vi "sub_main_F9P.vi"(8 "error in":errorcluster) -> (0 "error out":errorcluster)   [LabVIEW 2019]
panel:
  out "n":i32
  out "n2":i32
  out "n1":i32
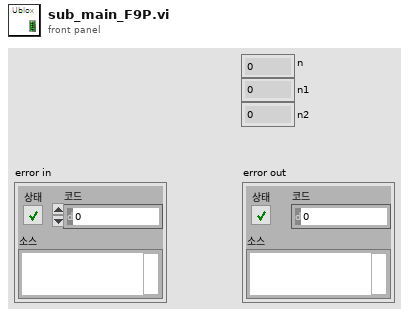
[diagram p1: front panel]
types:
  T1 = enum16{"GxDTM", "GxGBS", "GxGGA", "GxGLL", "GxGNS", "GxGRS", "GxGSA", "GxGST", "GxGSV", "GxRLM", "GxRMC", "GxTHS", "GxTXT", "GxVLW", "GxVTG", "GxZDA"}
  T2 = typedef "error_cluster.ctl" = cluster{"AGV":u8, "AGV Estop":u8, "Obstacle":u8, "Heading":u8, "Waypt":u8, "GNSS":u8, "VLP16":u8, "Cam":u8, "RPLidar":u8, "Joystick":u8, "IMU":u8}
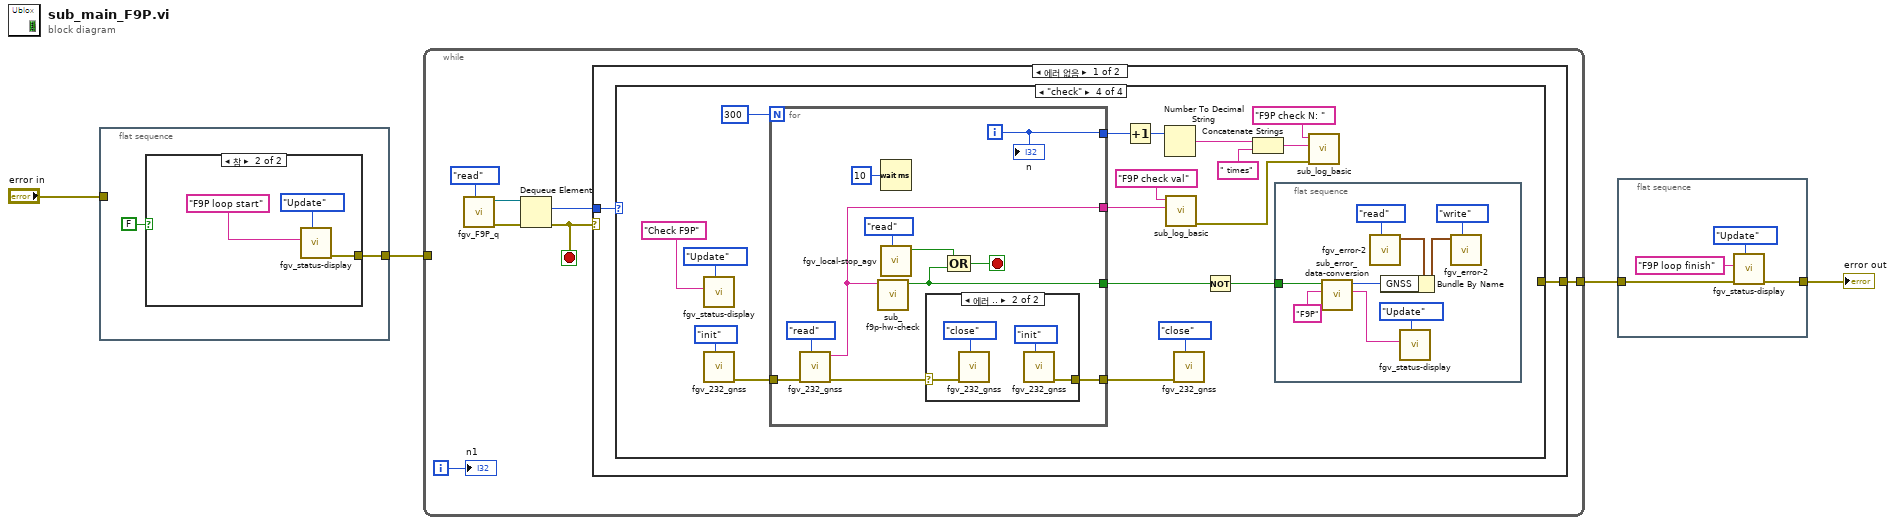
[diagram p0: block diagram]
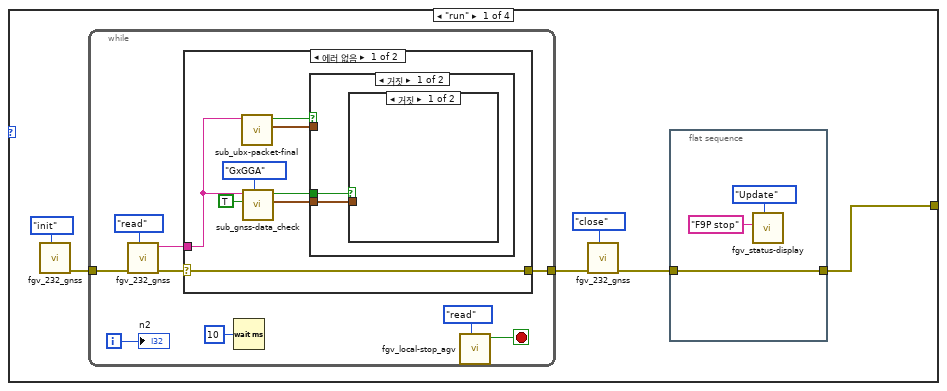
[diagram p3: hidden frame]
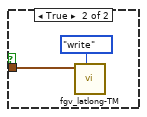
[diagram p4: hidden frame]
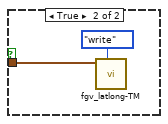
[diagram p5: hidden frame]
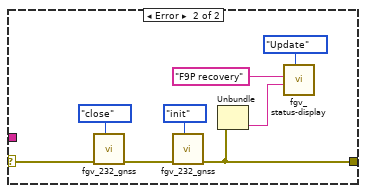
[diagram p6: hidden frame]
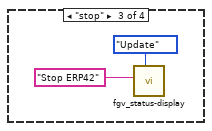
[diagram p8: hidden frame]
diagram:
  n1 = flat-sequence {
    tunnel: [w6] -> w1
    tunnel: "error in" -> [_]
    frame #0 {
      n2 = case shown="참" FALSE {
        tunnel: [_ w7] -> w6
        frame False {
        }
        frame True {
          n3 = call "fgv_status-display.vi"("Mode"=enum16{"Initial", "Update", "Clear"}."Update", "title"="F9P loop start" ("String in 1")) -> ("error out"=w7:errorcluster)  [unwired: 9 in]
        }
      }
    }
  }
  n4 = while {
    tunnel: w1 -> [_]
    tunnel: [w15] -> w2
    i -> [w14]
    stop <- w10 stop-if-true
    n5 = call "fgv_F9P_q.vi"("cmd"=enum16{"create", "write", "read", "close"}."read") -> ("error out"=w11:errorcluster, "queue out"=w12:refnum<queue>)  [unwired: 9 in]
    n6 = Dequeue Element(queue=w12, error in (no error)=w11) -> (element=w16:enum16{"run", "check", "stop"}, error out=w10:errorcluster)  [unwired: 1 in, 2 out]
    n7 = case shown="에러 없음" w10 {
      tunnel: w16 -> [w18 _]
      tunnel: [w17 _] -> w15
      frame No Error {
        n8 = case shown="\"check\"" w18 {
          tunnel: [w24 _ _ _] -> w17
          frame "run" {
            n9 = call "fgv_232_gnss.vi"("cmd"=enum16{"init", "read", "write", "close"}."init") -> ("error out"=w22:errorcluster)  [unwired: 8 in, 2 out]
            n10 = while {
              tunnel: [w31] -> w20
              tunnel: w22 -> [w33]
              i -> [w30]
              stop <- w35 stop-if-true
              n11 = call "fgv_232_gnss.vi"("cmd"=enum16{"init", "read", "write", "close"}."read", "error in"=w33) -> ("error out"=w28:errorcluster, "read_buffer"=w29:string)  [unwired: 7 in, 1 out]
              n12 = case shown="에러 없음" w28 {
                selector: w28 -> [w41 w57]
                tunnel: [w41 w52] -> w31
                tunnel: w29 -> [w43 _]
                frame No Error {
                  n13 = call "sub_ubx-packet-final.vi"("read_buffer"=w43) -> ("latlong"=w40:cluster{dbl, dbl}, "val"=w42:bool)  [unwired: 8 in, 1 out]
                  n14 = call "sub_gnss-data_check.vi"("sel"=T1."GxGGA", "log"=TRUE, "gnss str"=w43) -> ("LatLong"=w38:cluster{dbl, dbl}, "val"=w39:bool)  [unwired: 6 in, 1 out]
                  n15 = case shown="거짓" w42 {
                    tunnel: w40 -> [_ w49]
                    tunnel: w39 -> [w46 _]
                    tunnel: w38 -> [w45 _]
                    frame False {
                      n16 = case shown="거짓" w46 {
                        tunnel: w45 -> [_ w47]
                        frame False {
                        }
                        frame True {
                          n17 = call "fgv_latlong-TM.vi"("cmd"=enum16{"write", "read"}."write", "latlong"=w47) -> ()  [unwired: 8 in, 2 out]
                        }
                      }
                    }
                    frame True {
                      n18 = call "fgv_latlong-TM.vi"("cmd"=enum16{"write", "read"}."write", "latlong"=w49) -> ()  [unwired: 8 in, 2 out]
                    }
                  }
                }
                frame Error {
                  n19 = call "fgv_232_gnss.vi"("cmd"=enum16{"init", "read", "write", "close"}."close", "error in"=w57) -> ("error out"=w53:errorcluster)  [unwired: 7 in, 2 out]
                  n20 = call "fgv_232_gnss.vi"("cmd"=enum16{"init", "read", "write", "close"}."init", "error in"=w53) -> ("error out"=w52:errorcluster)  [unwired: 7 in, 2 out]
                  n21 = Unbundle(w52) -> ("source"=w51:string)  [unwired: 2 out]
                  n22 = call "fgv_status-display.vi"("Mode"=enum16{"Initial", "Update", "Clear"}."Update", "detail"=w51, "title"="F9P recovery" ("String in 1")) -> ()  [unwired: 8 in, 1 out]
                }
              }
              n23 = Wait (ms)(milliseconds to wait=u32 10 ("대기 시간 (ms)")) -> ()  [unwired: 1 out]
              n24 = call "fgv_local-stop_agv.vi"("cmd"=enum16{"ini", "read", "stop"}."read") -> ("stop status"=w35:bool)  [unwired: 10 in]
              "n2" <- w30
            }
            n25 = call "fgv_232_gnss.vi"("cmd"=enum16{"init", "read", "write", "close"}."close", "error in"=w20) -> ("error out"=w19:errorcluster)  [unwired: 7 in, 2 out]
            n26 = flat-sequence {
              tunnel: [w25] -> w24
              tunnel: w19 -> [w25]
              frame #0 {
                n27 = call "fgv_status-display.vi"("Mode"=enum16{"Initial", "Update", "Clear"}."Update", "title"="F9P stop" ("String in 1")) -> ()  [unwired: 9 in, 1 out]
              }
            }
          }
          frame Default {
          }
          frame "stop" {
            n28 = call "fgv_status-display.vi"("Mode"=enum16{"Initial", "Update", "Clear"}."Update", "title"="Stop ERP42" ("String in")) -> ()  [unwired: 9 in, 1 out]
          }
          frame "check" {
            n29 = call "fgv_status-display.vi"("Mode"=enum16{"Initial", "Update", "Clear"}."Update", "title"="Check F9P" ("String in")) -> ()  [unwired: 9 in, 1 out]
            n30 = call "fgv_232_gnss.vi"("cmd"=enum16{"init", "read", "write", "close"}."init") -> ("error out"=w74:errorcluster)  [unwired: 8 in, 2 out]
            n31 = for {
              N: 300 -> [_]
              tunnel: w74 -> [w96]
              tunnel: [w88] -> w72
              tunnel: [w94] -> w71
              tunnel: [w91] -> w67
              tunnel: [w90] -> w66
              i -> [w91]
              stop <- w92 stop-if-true
              n32 = call "fgv_232_gnss.vi"("cmd"=enum16{"init", "read", "write", "close"}."read", "error in"=w96) -> ("error out"=w89:errorcluster, "read_buffer"=w90:string)  [unwired: 7 in, 1 out]
              n33 = call "sub_f9p-hw-check.vi"("GNSS str"=w90) -> ("val"=w94:bool)  [unwired: 10 in]
              n34 = Wait (ms)(milliseconds to wait=u32 10 ("대기 시간 (ms)")) -> ()  [unwired: 1 out]
              n35 = call "fgv_local-stop_agv.vi"("cmd"=enum16{"ini", "read", "stop"}."read") -> ("stop status"=w93:bool)  [unwired: 10 in]
              n36 = case shown="에러 .." w89 {
                selector: w89 -> [w99 w102]
                tunnel: [w99 w100] -> w88
                frame No Error {
                }
                frame Error {
                  n37 = call "fgv_232_gnss.vi"("cmd"=enum16{"init", "read", "write", "close"}."close", "error in"=w102) -> ()  [unwired: 7 in, 3 out]
                  n38 = call "fgv_232_gnss.vi"("cmd"=enum16{"init", "read", "write", "close"}."init") -> ("error out"=w100:errorcluster)  [unwired: 8 in, 2 out]
                }
              }
              n39 = Compound Arithmetic op=OR ("복합 연산")(w93, w94) -> (w92:bool)
              "n" <- w91
            }
            n40 = Increment(x=w67) -> (x+1=w70:i32)
            n41 = Number To Decimal String(number=w70) -> (decimal integer string=w69:string)  [unwired: 1 in]
            n42 = call "sub_log_basic.vi"("desc"=w66, "Title"="F9P check val") -> ("error out"=w62:errorcluster)  [unwired: 9 in]
            n43 = call "fgv_232_gnss.vi"("cmd"=enum16{"init", "read", "write", "close"}."close", "error in"=w72) -> ()  [unwired: 7 in, 3 out]
            n44 = Not(x=w71) -> (.not. x?=w61:bool)
            n45 = Concatenate Strings(w69, " times" ("문자열")) -> (w64:string)
            n46 = flat-sequence {
              tunnel: w61 -> [w82]
              frame #0 {
                n47 = call "sub_error_data-conversion.vi"("name"="F9P", "error status"=w82) -> ("check result string"=w79:string, "error conversion out"=w87:u8)  [unwired: 8 in]
                n48 = call "fgv_error-2.vi"("cmd"=enum16{"init", "read", "write"}."read") -> ("Error cluster out"=w86:T2)  [unwired: 9 in, 1 out]
                n49 = Bundle By Name(cluster=w86, "GNSS"=w87) -> (w85:T2)
                n50 = call "fgv_status-display.vi"("Mode"=enum16{"Initial", "Update", "Clear"}."Update", "title"=w79) -> ()  [unwired: 9 in, 1 out]
                n51 = call "fgv_error-2.vi"("cmd"=enum16{"init", "read", "write"}."write", "Error cluster"=w85) -> ()  [unwired: 8 in, 2 out]
              }
            }
            n52 = call "sub_log_basic.vi"("error in"=w62, "desc"=w64, "Title"="F9P check N: ") -> ()  [unwired: 8 in, 1 out]
          }
        }
      }
      frame Error {
      }
    }
    "n1" <- w14
  }
  n53 = flat-sequence {
    tunnel: [w105] -> w3
    tunnel: w2 -> [w104]
    frame #0 {
      n54 = call "fgv_status-display.vi"("Mode"=enum16{"Initial", "Update", "Clear"}."Update", "error in"=w104, "title"="F9P loop finish" ("String in 1")) -> ("error out"=w105:errorcluster)  [unwired: 8 in]
    }
  }
  "error out" <- w3
